vi "RRR_Forward_Kinematics_2025.vi"() -> ()   [LabVIEW 2020]
panel:
  in  "Claw Value":dbl(slide)=1.0 scale=0.0..1.0
  in  "Claw Angle":dbl
  in  "Base position  Y":dbl
  in  "Base position X":dbl
  in  "Scale Factor":dbl(slide)=0.7 scale=0.5..1.0
  out "RRR - Forward Kinematics Visual":picture
  in  "Add details":bool=TRUE
  in  "Light Direction":dbl(knob)=5.611498737356196 scale format="%#.1f"
  in  "Colors":T1={"Joint 1"=16750848, "Arm 1"=16764006, "Joint 2"=26316, "Arm B"=6723993, "Joint 4"=16724787, "Claw"=16776960, "Joint 3"=26316, "Arm C"=6723993}
  out "TCP_Y":dbl
  out "Joint2_Y":dbl
  out "Joint1_Y":dbl
  out "TCP_X":dbl=100.0
  out "Joint2_X":dbl=80.0
  out "Joint1_X":dbl=50.0
  in  "Arm 3":dbl=20.0
  in  "Joint 3":dbl
  out "RRR - Forward Kinematics":cluster{dbl[], dbl[]}(graph)={[0.0, 50.0, 80.0, 100.0], [0.0, 0.0, 0.0, 0.0]}
  in  "Joint 2":dbl
  in  "Joint 1":dbl
  in  "Arm 2":dbl=30.0
  in  "Arm 1":dbl=50.0
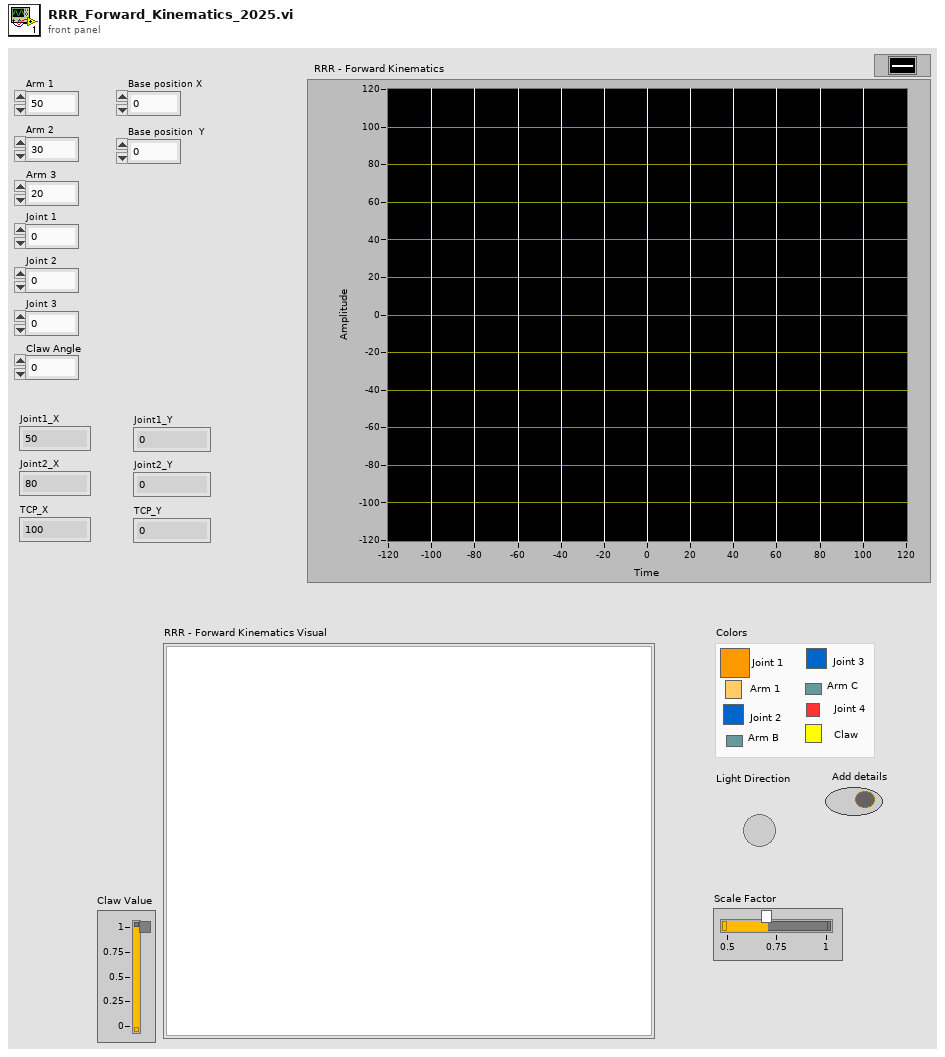
[diagram p1: front panel]
types:
  T1 = cluster{"Joint 1":u32, "Arm 1":u32, "Joint 2":u32, "Arm B":u32, "Joint 4":u32, "Claw":u32, "Joint 3":u32, "Arm C":u32}
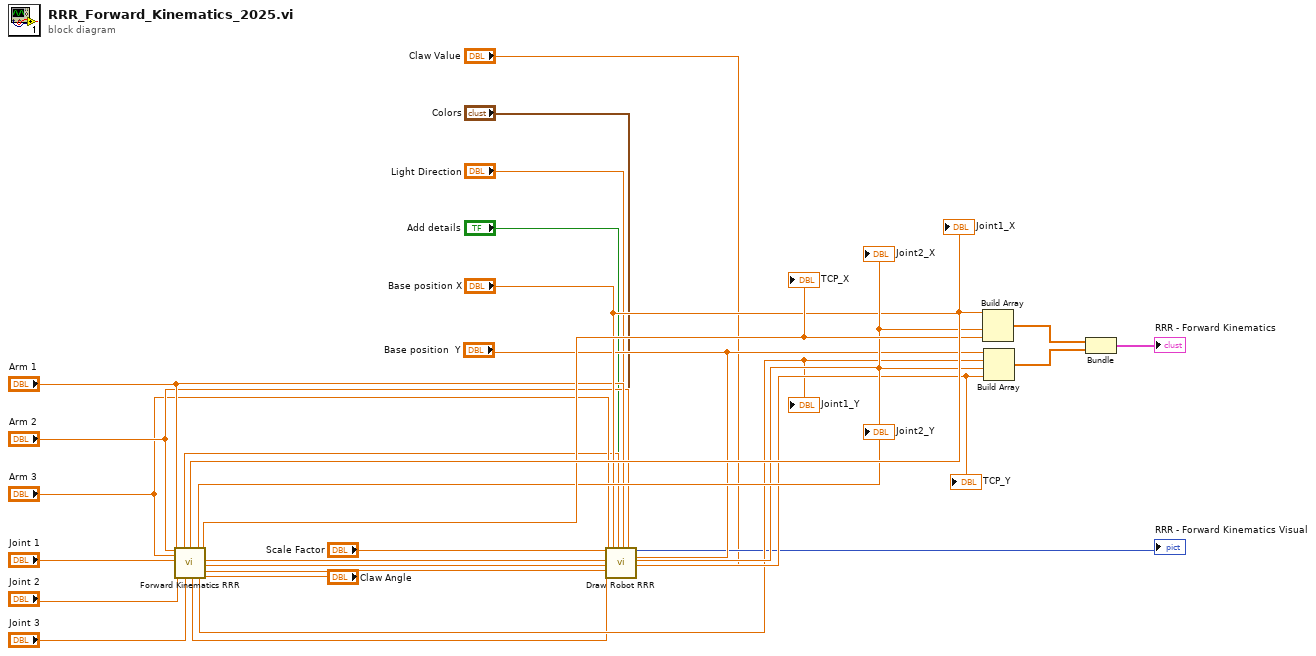
[diagram p0: block diagram]
diagram:
  n1 = call "Forward Kinematics RRR.vi"("Arm in"="Arm 2", "Arm 3"="Arm 3", "Joint 1"="Joint 1", "Joint in"="Joint 2", "Joint 3"="Joint 3", "Arm 1"="Arm 1", "Claw Angle"="Claw Angle") -> ("Numeric"=w7:dbl, "x1"=w26:dbl, "Numeric 2"=w10:dbl, "x2"=w20:dbl, "Numeric 3"=w13:dbl, "x_final"=w21:dbl, "y1"=w17:dbl, "y2"=w19:dbl, "y_final"=w18:dbl, "Numeric 4"=w16:dbl)  [unwired: 3 in]
  "Joint1_X" <- w26
  "Joint2_X" <- w20
  "TCP_X" <- w21
  "Joint1_Y" <- w17
  "Joint2_Y" <- w19
  "TCP_Y" <- w18
  n2 = call "Draw Robot RRR.vi"("Scale Factor"="Scale Factor", "Base position  Y"="Base position  Y", "Claw Value"="Claw Value", "Numeric 4"=w16, "Arm 3"="Arm 3", "Numeric 3"=w13, "Base position X"="Base position X", "Numeric 2"=w10, "Add details"="Add details", "Numeric"=w7, "Light Direction"="Light Direction", "Arm 1"="Arm 1", "Colors"="Colors", "Arm in"="Arm 2") -> ("Picture Out"=→"RRR - Forward Kinematics Visual":picture)  [unwired: 5 in]
  n3 = Build Array("Base position X", w26, w20, w21) -> (w25:dbl[])
  n4 = Build Array("Base position  Y", w17, w19, w18) -> (w24:dbl[])
  n5 = Bundle(w25, w24) -> (→"RRR - Forward Kinematics":cluster{dbl[], dbl[]})  [unwired: 1 in]
